vi "AskUserPass.vi"(5 "port":string) -> (2 "Port out":string)   [LabVIEW 2022 SP3]
panel:
  in  "password":string
  in  "username":string
  in  "append":bool caption="Cancel"
  in  "once":bool caption="OK2"
  # "You have not stored a username/password in preferences for this IP.  What are the username and password?"
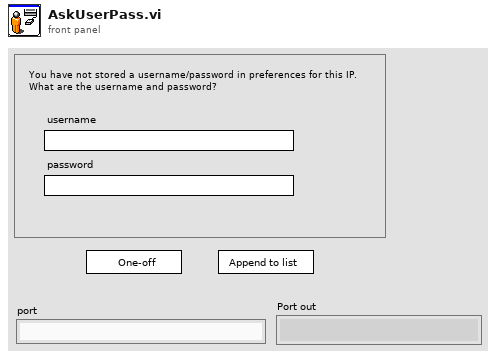
[diagram p1: front panel]
types:
  T1 = cluster{"IP Address":string, "Username":string, "password":string}
  T2 = cluster{"IP Address":string, "username":string, "password":string}
  T3 = typedef "Preferences.ctl" = cluster{"python":string, "arduino CLI":path, "pythonCodes":cluster{"pythonCode":path, "Color":u32}[], "FontSize":u8, "Text Colors":cluster{"Quote":u32, "function":u32, "Python":u32, "Comment":u32, "Triple Quote":u32, "Text":u32}, "SSH Logins":cluster{"IP Address":string, "Username":string, "password":string}[], "packet size":u8}
  T4 = cluster{"IP Address":string, "Username":string, "password":string}[]
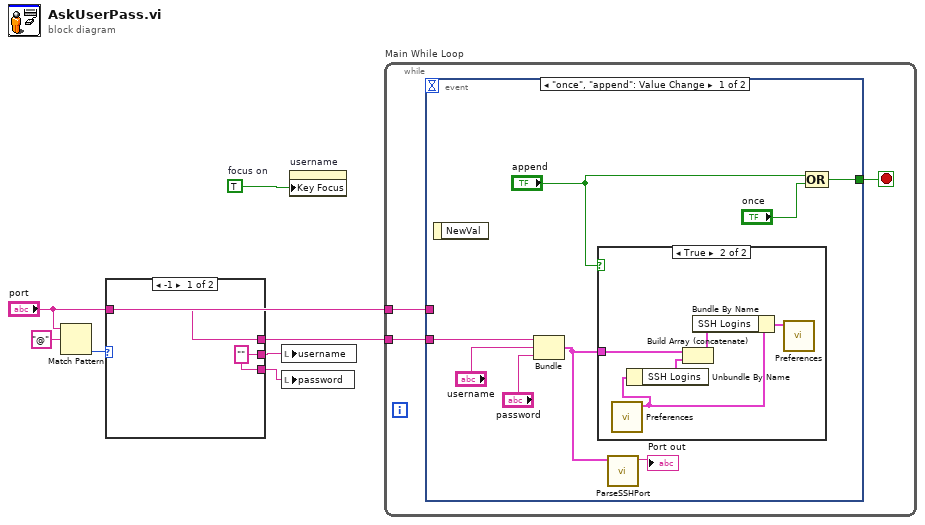
[diagram p0: block diagram]
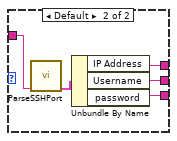
[diagram p2: hidden frame]
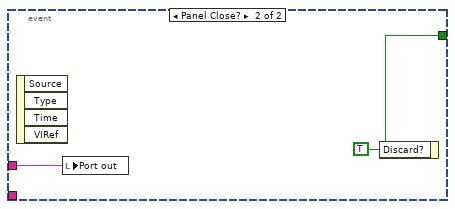
[diagram p4: hidden frame]
diagram:
  w7 = TRUE  # focus on
  n1 = Match Pattern(string="port", regular expression="@") -> (offset past match=w1:i32)  [unwired: 1 in, 3 out]
  n2 = case shown="-1" w1 {
    tunnel: [w8 w13] -> w6
    tunnel: [w8 w12] -> w5
    tunnel: [w9 w11] -> w4
    tunnel: "port" -> [w9 w10]
    frame -1 {
      w8 = "" ("Username")
    }
    frame Default {
      n3 = call "ParseSSHPort.vi"("String in"=w10) -> ("port"=w14:T1)  [unwired: 8 in, 2 out]
      n4 = Unbundle By Name(w14) -> ("IP Address"=w11:string, "Username"=w13:string, "password"=w12:string)
    }
  }
  n5 = local write "username"(w6) -> ()
  n6 = local write "password"(w5) -> ()
  n7 = property on="username" class="Str"("Key Focus"=w7) -> ()  [unwired: 2 in, 2 out]
  n8 = while "Main While Loop" {
    tunnel: w4 -> [w17]
    tunnel: "port" -> [w15]
    stop <- w16 stop-if-true
    n9 = event shown="[0] \"once\", \"append\": Value Change" {
      selector: _ -> [_ _]
      dyn-events: _ -> [_ _]
      timeout: _ -> [_ _]
      tunnel: [w25 w32] -> w16
      tunnel: w17 -> [w22 _]
      tunnel: w15 -> [_ w31]
      event "once", "append": Value Change {
        n10 = event-data() -> ()  [unwired: 1 in, 1 out]
        n11 = Bundle("IP Address"=w22, "username"="username", "password"="password") -> (w19:T2)  [unwired: 1 in]
        n12 = case shown="True" "append" {
          tunnel: w19 -> [_ w30]
          frame False {
          }
          frame True {
            n13 = call "Preferences.vi"() -> ("Preferences out"=w28:T3)  [unwired: 10 in, 1 out]
            n14 = Unbundle By Name(w28) -> ("SSH Logins"=w29:T4)
            n15 = Build Array (concatenate)(w30, w29) -> (w27:T4)
            n16 = Bundle By Name(cluster=w28, "SSH Logins"=w27) -> (w26:T3)
            n17 = call "Preferences.vi"("Preferences in"=w26) -> ()  [unwired: 9 in, 2 out]
          }
        }
        n18 = call "ParseSSHPort.vi"("SSH Login"=w19) -> ("Full String out"=→"Port out":string)  [unwired: 8 in, 2 out]
        n19 = Compound Arithmetic op=OR("append", "once") -> (w25:bool)
      }
      event Panel Close? {
        w32 = TRUE ("Discard?")
        n20 = event-data() -> ()  [unwired: 1 in, 4 out]
        n21 = local write "Port out"(w31) -> ()
        n22 = event-data("Discard?"=w32) -> ()  [unwired: 1 in, 1 out]
      }
    }
  }
